vi "(BASVR) Manage Iterations.vi"(4 "Loop's Channel List":u8[](array[numeric]), 5 "Current Channel":u8, 7 "MI Cluster":T1) -> (0 "Continue current graph?":bool, 1 "Finish AVS Loop?":bool, 2 "group name out":string, 3 "Logging File Refnum":refnum<k34>)   [LabVIEW 2023]
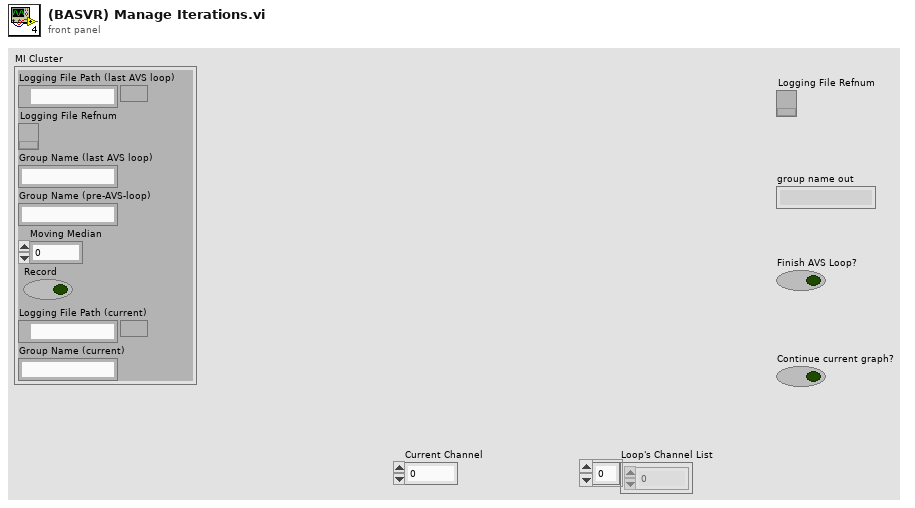
[diagram p1: front panel]
types:
  T1 = cluster{"Logging File Path (last AVS loop)":path, "Logging File Refnum":refnum<k34>, "Group Name (last AVS loop)":string, "Group Name (pre-AVS-loop)":string, "Moving Median":u8, "Record":bool, "Logging File Path (current)":path, "Group Name (current)":string}
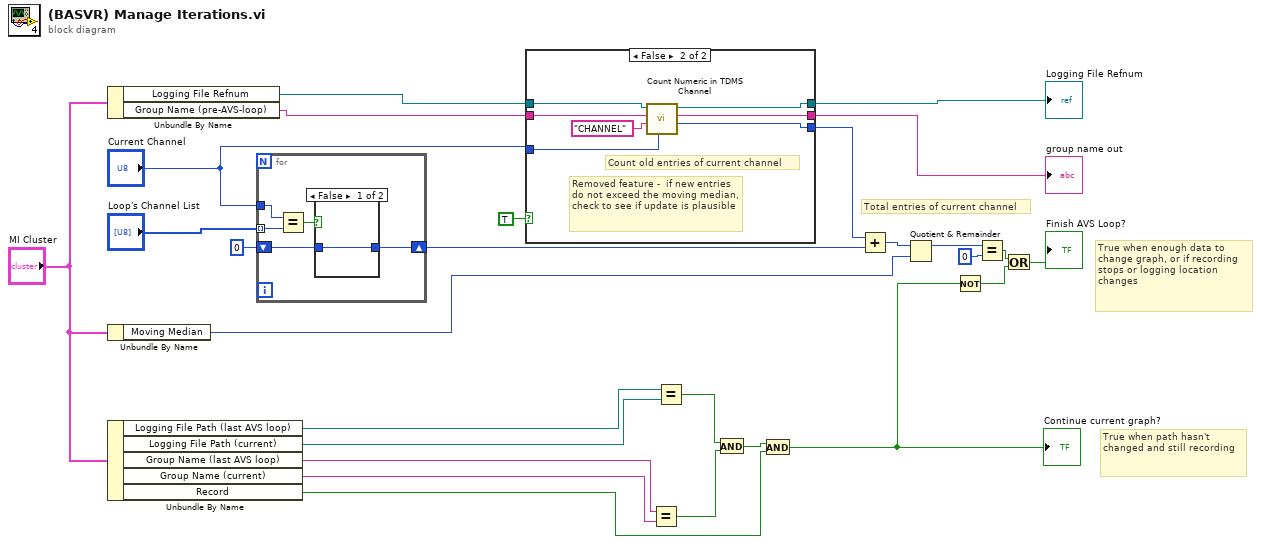
[diagram p0: block diagram]
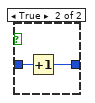
[diagram p2: hidden frame]
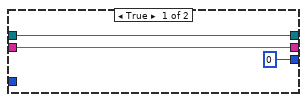
[diagram p3: hidden frame]
diagram:
  # "True when path hasn't changed and still recording"
  # "Total entries of current channel"
  # "True when enough data to change graph, or if recording stops or logging location changes"
  n1 = Unbundle By Name("MI Cluster") -> ("Logging File Refnum"=w10:refnum<k34>, "Group Name (pre-AVS-loop)"=w9:string)
  n2 = Unbundle By Name("MI Cluster") -> ("Moving Median"=w8:u8)
  n3 = Unbundle By Name("MI Cluster") -> ("Logging File Path (last AVS loop)"=w7:path, "Logging File Path (current)"=w6:path, "Group Name (last AVS loop)"=w4:string, "Group Name (current)"=w3:string, "Record"=w5:bool)
  n4 = for {
    tunnel: "Loop's Channel List" -> [w28] mode=indexing
    shift-right: [w31] -> w21
    shift-left: 0 -> [w30]
    tunnel: "Current Channel" -> [w29]
    n5 = Equal?(x=w29, y=w28) -> (x = y?=w32:bool)
    n6 = case shown="False" w32 {
      tunnel: [w33 w35] -> w31
      tunnel: w30 -> [w33 w34]
      frame False {
      }
      frame True {
        n7 = Increment(x=w34) -> (x+1=w35:i32)
      }
    }
  }
  n8 = case shown="False" TRUE {
    tunnel: w10 -> [w38 w44]
    tunnel: w9 -> [w37 w43]
    tunnel: [w37 w42] -> w11
    tunnel: "Current Channel" -> [_ w41]
    tunnel: [w38 w40] -> w12
    tunnel: [0 w39] -> w13
    frame True {
    }
    frame False {
      # "Removed feature -  if new entries do not exceed the moving median, check to see if update is plausible"
      # "Count old entries of current channel"
      n9 = call "Count Numeric in TDMS Channel.vi"("CHANNEL"=w41, "Channel Name"="CHANNEL", "Group Name"=w43, "Refnum in"=w44) -> ("Count"=w39:i32, "group name out"=w42:string, "Refnum out"=w40:refnum<k34>)  [unwired: 4 in, 1 out]
    }
  }
  "Logging File Refnum" <- w12
  "group name out" <- w11
  n10 = Equal?(x=w4, y=w3) -> (x = y?=w26:bool)
  n11 = Equal?(x=w7, y=w6) -> (x = y?=w25:bool)
  n12 = And(x=w25, y=w26) -> (x .and. y?=w24:bool)
  n13 = And(x=w24, y=w5) -> (x .and. y?=w27:bool)
  "Continue current graph?" <- w27
  n14 = Add(x=w13, y=w21) -> (x+y=w14:i32)
  n15 = Quotient & Remainder(x=w14, y=w8) -> (x-y*floor(x/y)=w15:i32)  [unwired: 1 out]
  n16 = Not(x=w27) -> (.not. x?=w18:bool)
  n17 = Equal?(x=w15, y=0) -> (x = y?=w17:bool)
  n18 = Or(x=w17, y=w18) -> (x .or. y?=→"Finish AVS Loop?":bool)
